vi "resultsColumnsPlugins.vi"(10 "chValuesIn":string[](array[string]), 11 "chNamesIn":string[](array[string])) -> (2 "chValuesOut":string[](array[string]), 3 "chNamesOut":string[](array[string]))   [LabVIEW 2020]
uses:
  Globals/Dynamic_call_global.ph.vi
  Globals/Meas_global.vi
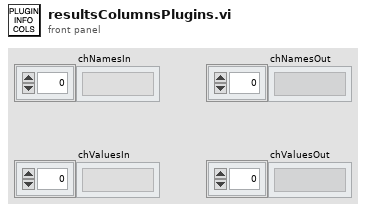
[diagram p1: front panel]
types:
  T1 = typedef "Post_Process.ctl" = enum16{"Take New Data", "Post Process Raw Data File"}
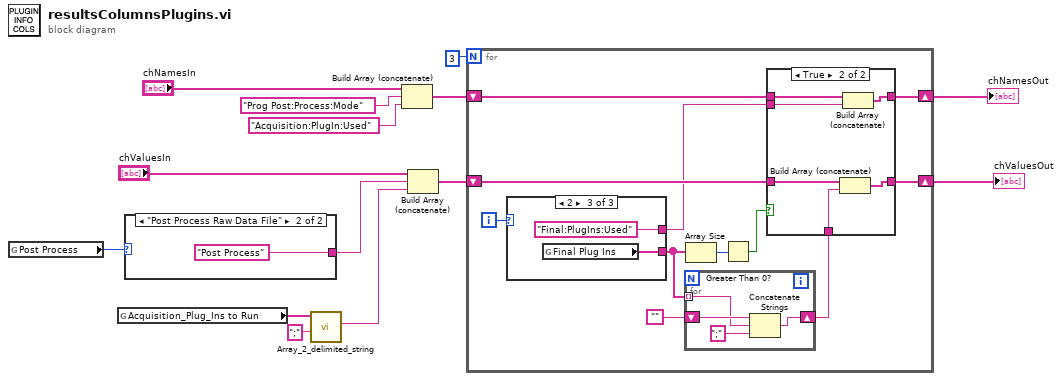
[diagram p0: block diagram]
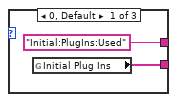
[diagram p3: hidden frame]
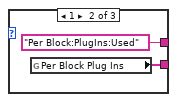
[diagram p4: hidden frame]
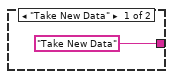
[diagram p5: hidden frame]
diagram:
  n1 = global read "Meas_global.vi" "Post Process"() -> (w14:T1)
  n2 = global read "Meas_global.vi" "Acquisition_Plug_Ins to Run"() -> (w9:string[])
  n3 = case shown="\"Post Process Raw Data File\"" w14 {
    tunnel: ["Take New Data" "Post Process"] -> w2
    frame "Take New Data" {
    }
    frame "Post Process Raw Data File" {
    }
  }
  n4 = call "Array_2_delimited_string.vi"("delimiter (Tab)"=";", "Array of Strings"=w9) -> ("delimited string"=w10:string)  [unwired: 9 in]
  n5 = Build Array (concatenate)("chNamesIn", "Prog Post:Process:Mode" ("Input Element"), "Acquisition:PlugIn:Used" ("Input Element")) -> (w7:string[])
  n6 = Build Array (concatenate)("chValuesIn", w2, w10) -> (w4:string[])
  n7 = for {
    N: 3 -> [_]
    shift-right: [w22] -> w13
    shift-left: w4 -> [w23]
    shift-right: [w18] -> w12
    shift-left: w7 -> [w19]
    i -> [w26]
    n8 = case shown="2" w26 {
      tunnel: [w37 w39 w41] -> w20
      tunnel: ["Initial:PlugIns:Used" ("Input Element") "Per Block:PlugIns:Used" ("Input Element") "Final:PlugIns:Used" ("Input Element")] -> w17
      frame 0, Default {
        n9 = global read "Dynamic_call_global.ph.vi" "Initial Plug Ins"() -> (w37:string[])
      }
      frame 1 {
        n10 = global read "Dynamic_call_global.ph.vi" "Per Block Plug Ins"() -> (w39:string[])
      }
      frame 2 {
        n11 = global read "Dynamic_call_global.ph.vi" "Final Plug Ins"() -> (w41:string[])
      }
    }
    n12 = for {
      tunnel: w20 -> [w42] mode=indexing
      shift-right: [w43] -> w21
      shift-left: "" -> [w45]
      n13 = Concatenate Strings(w45, w42, ";" ("string")) -> (w43:string)
    }
    n14 = Array Size(array=w20) -> (size(s)=w25:i32)
    n15 = Greater Than 0?(x=w25) -> (x > 0?=w24:bool)
    n16 = case shown="True" w24 {
      tunnel: w23 -> [w29 w35]
      tunnel: [w29 w34] -> w22
      tunnel: w21 -> [_ w33]
      tunnel: w19 -> [w28 w32]
      tunnel: [w28 w31] -> w18
      tunnel: w17 -> [_ w30]
      frame False {
      }
      frame True {
        n17 = Build Array (concatenate)(w35, w33) -> (w34:string[])
        n18 = Build Array (concatenate)(w32, w30) -> (w31:string[])
      }
    }
  }
  "chValuesOut" <- w13
  "chNamesOut" <- w12
